vi "NI9205_UI_LinearLoadCell.vi"() -> ()   [LabVIEW 2020]
uses:
  TYPEDEF/NI9205_TD_QueueSaveData.ctl
  TYPEDEF/NI9205_TD_Method.ctl
panel:
  out "LastSaved":string
  in  "MaximumSampleRate?":bool
  in  "SampleRate":dbl=1000.0 format="%0.2f"
  out "queueDataToSave":refnum<queue>
  in  "ClearData":bool
  in  "Save Now":bool
  out "Data size":i32
  in  "Nomefile_txt":string
  in  "file path":path
  out "Meter [kN]":dbl(knob) scale=0.0..100.0
  out "Waveform Graph 2":dbl[](graph)
  out "V":dbl
  out "LC (kN)":dbl
  in  "q":dbl=2.15875
  in  "gain":dbl=-22.26172
  out "Waveform Graph":waveform(dbl)[](graph)
  in  "Stop":bool
  in  "Start":bool
  in  "Number of Samples":i32=100
  in  "Channels NI9205":tag="cDAQ2Mod2/ai6"
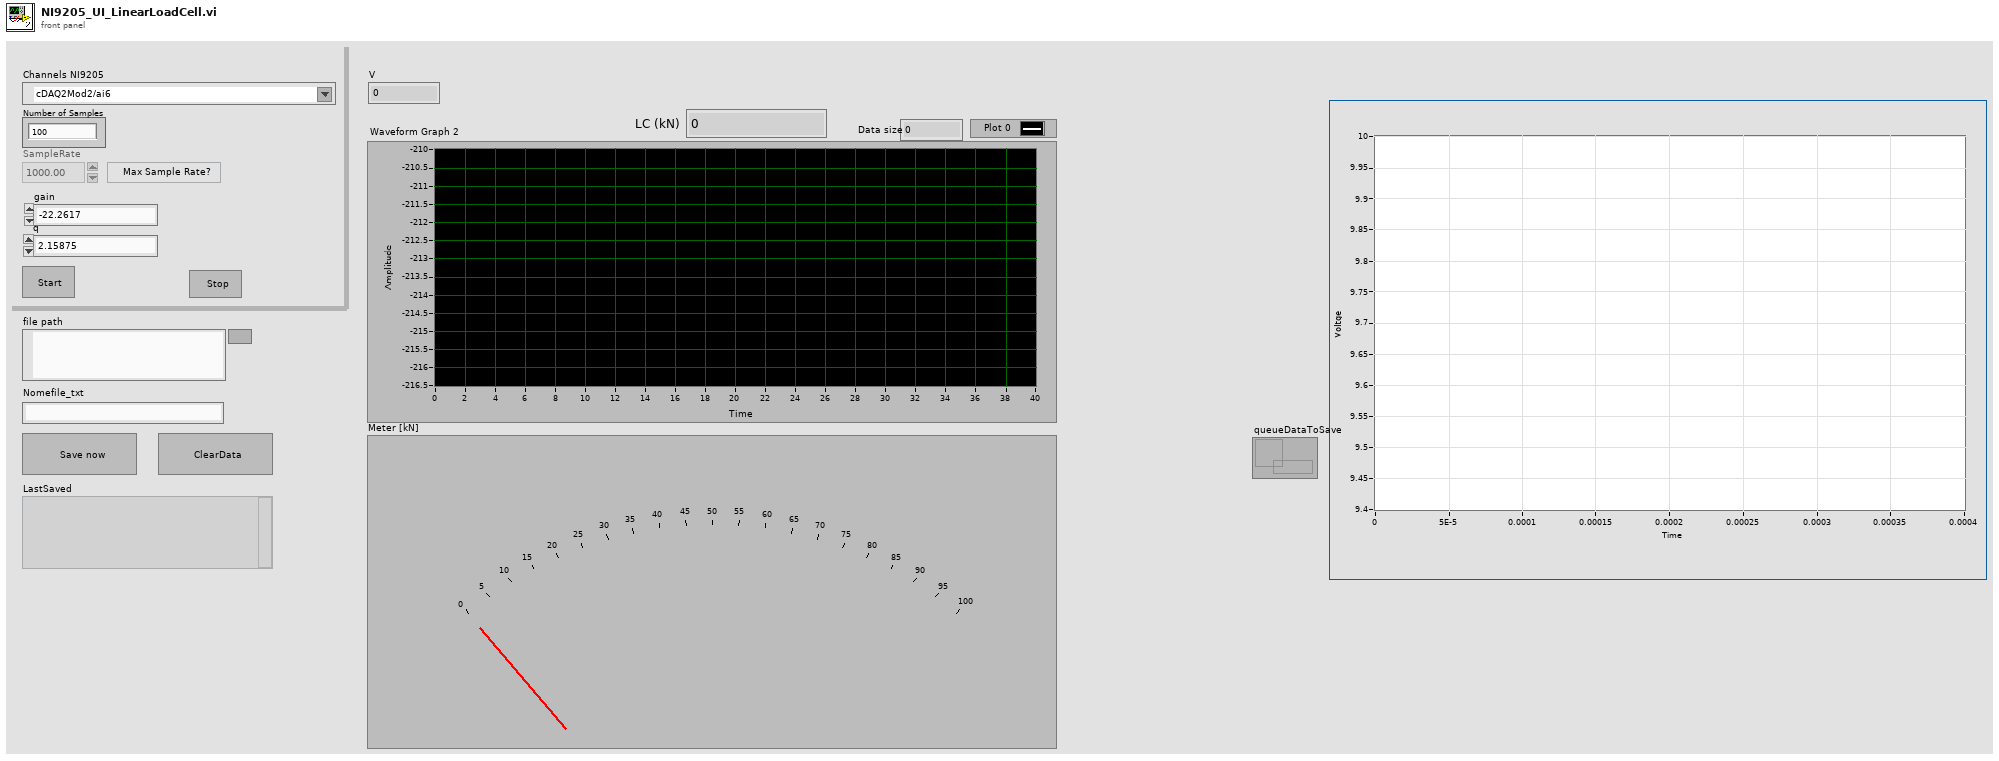
[diagram p1: front panel]
types:
  T1 = enum8{"Enabled", "Disabled", "Disabled and Grayed Out"}
  T2 = typedef "NI9205_TD_QueueSaveData.ctl" = cluster{"TimeData":timestamp[], "Ydata":dbl[], "AutoSaved?":bool}
  T3 = typedef "NI9205_TD_Method.ctl" = enum16{"NO_OP", "INIT", "SET", "GET", "CLOSE"}
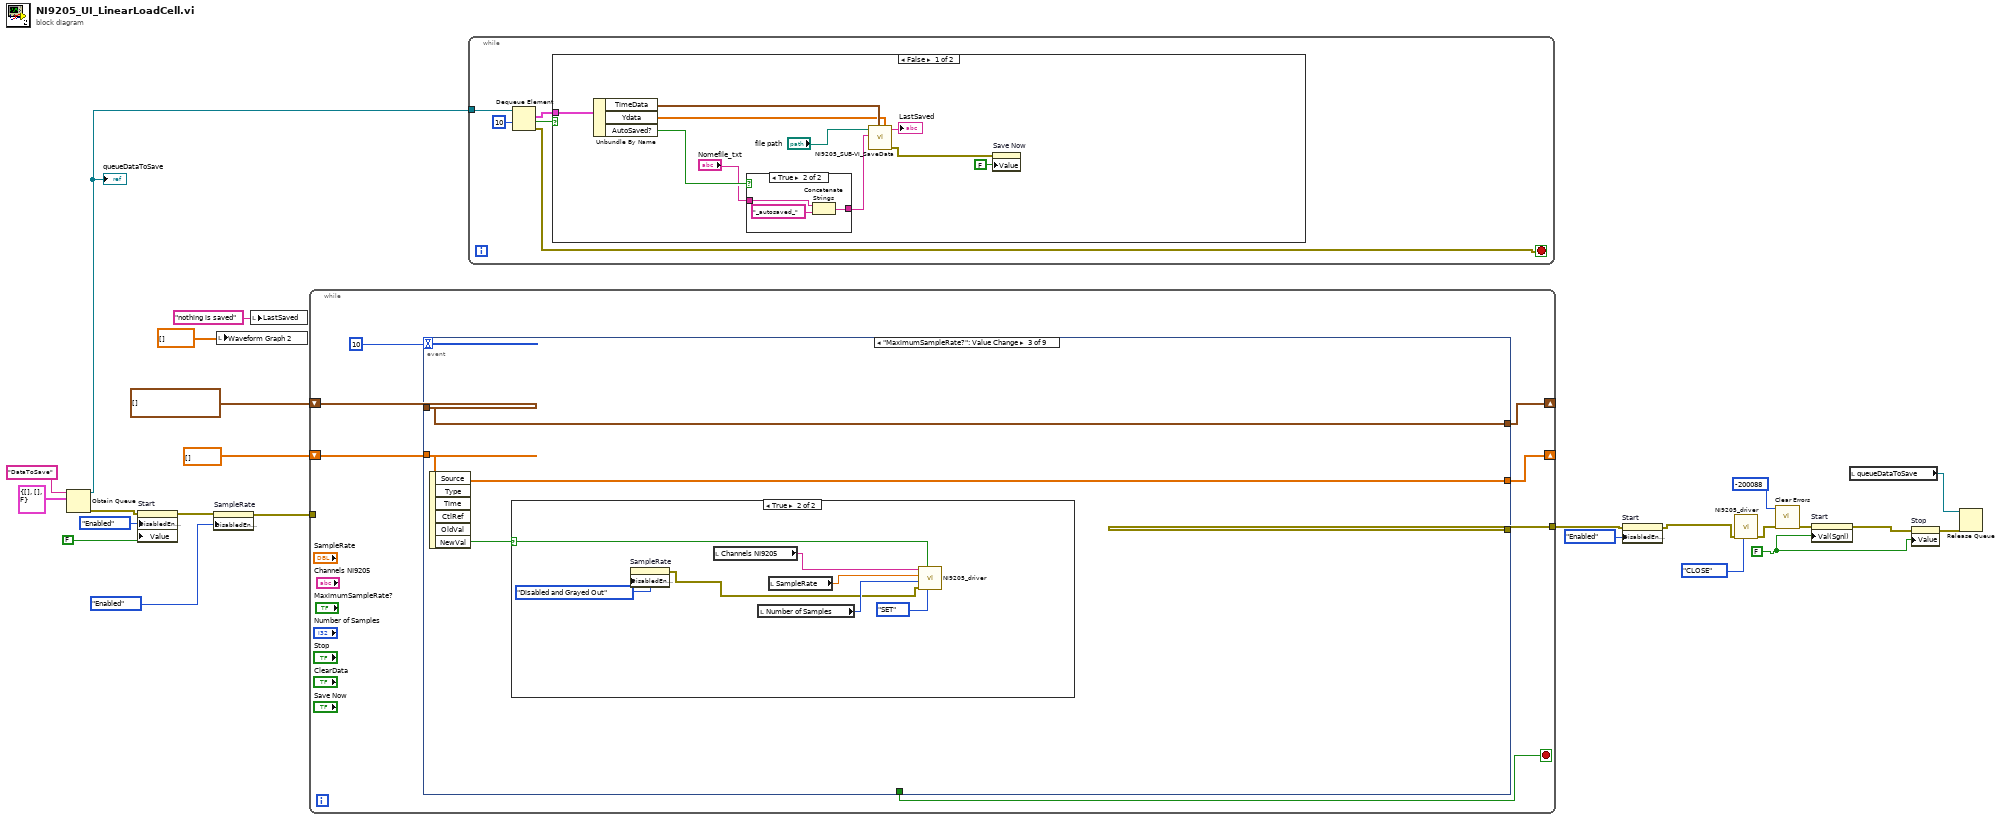
[diagram p0: block diagram]
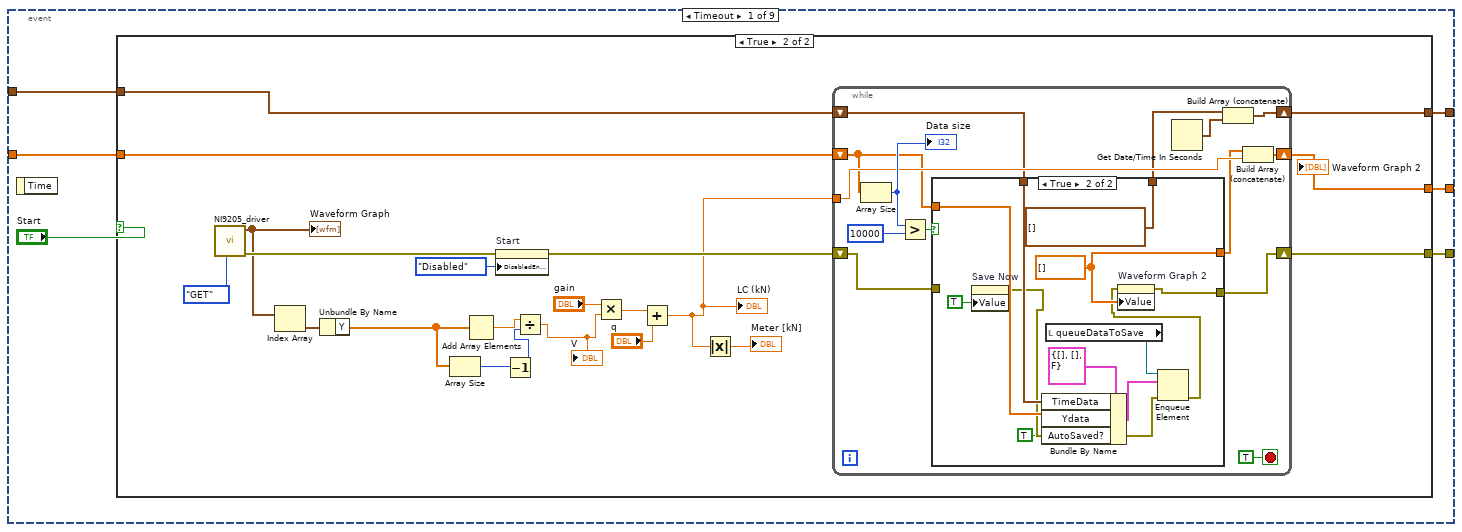
[diagram p4: hidden frame]
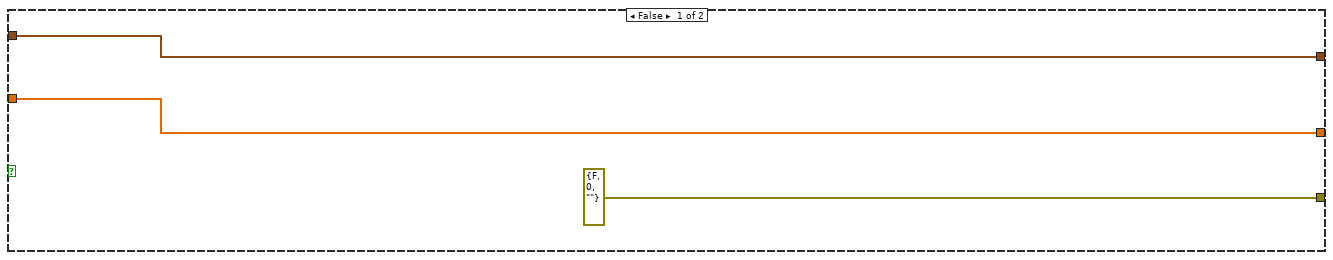
[diagram p5: hidden frame]
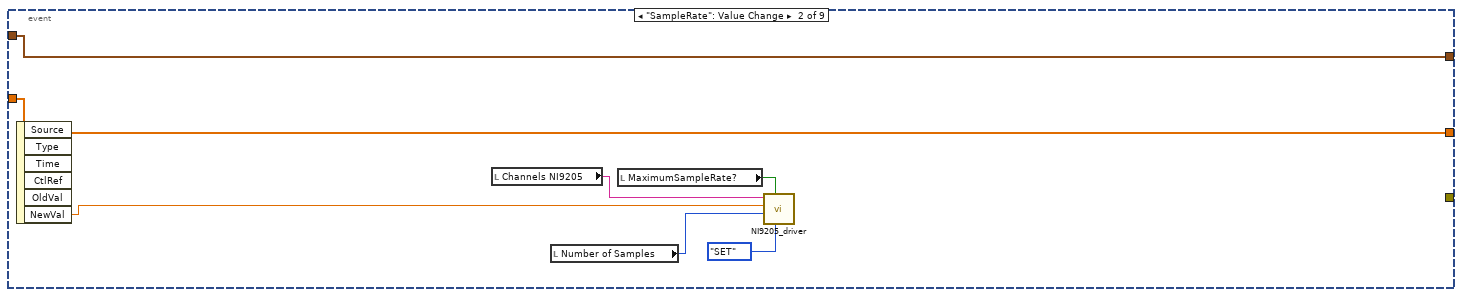
[diagram p7: hidden frame]
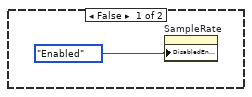
[diagram p8: hidden frame]
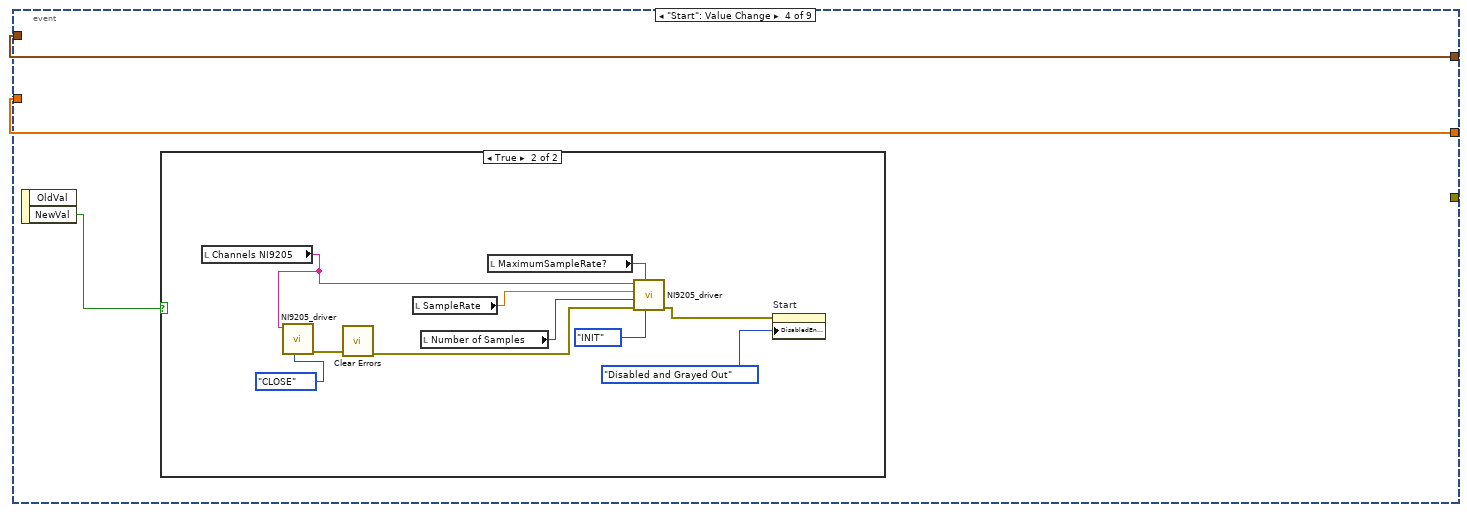
[diagram p9: hidden frame]
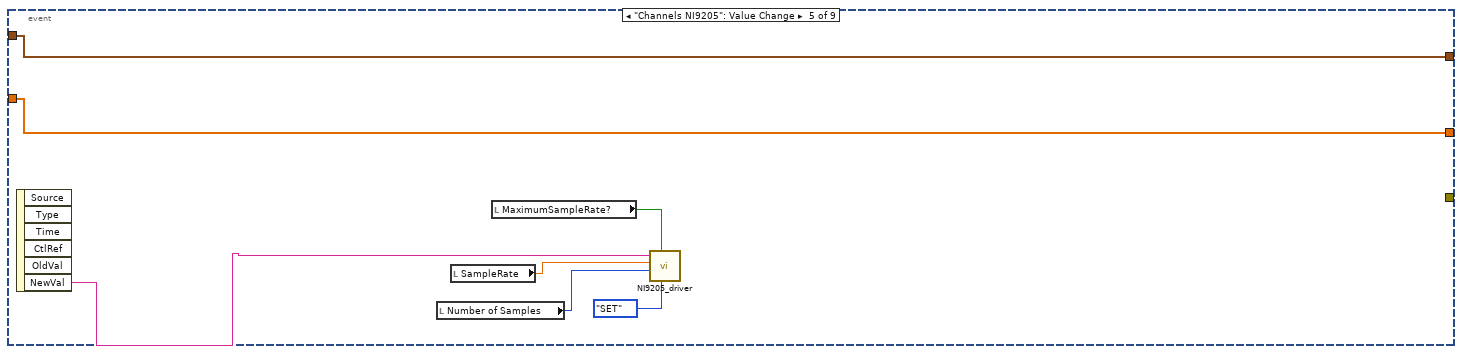
[diagram p11: hidden frame]
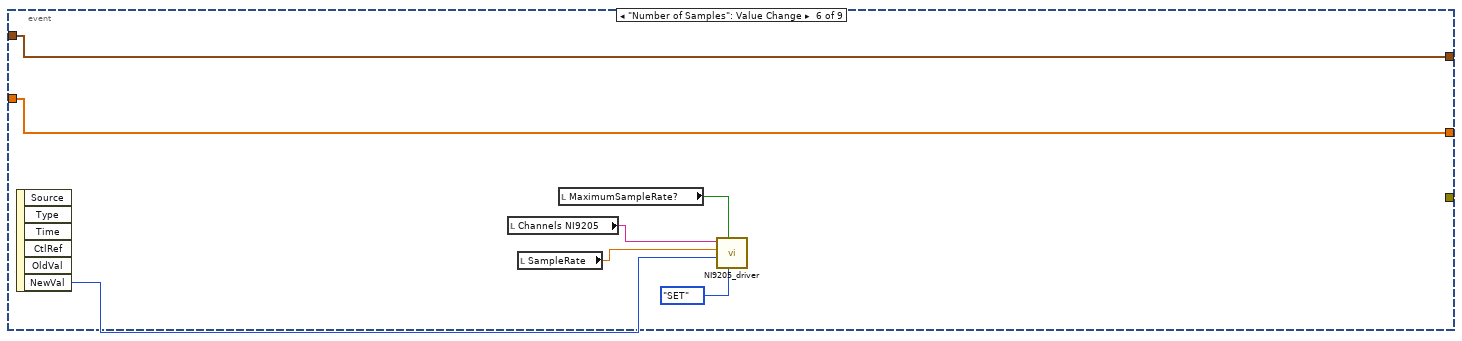
[diagram p12: hidden frame]
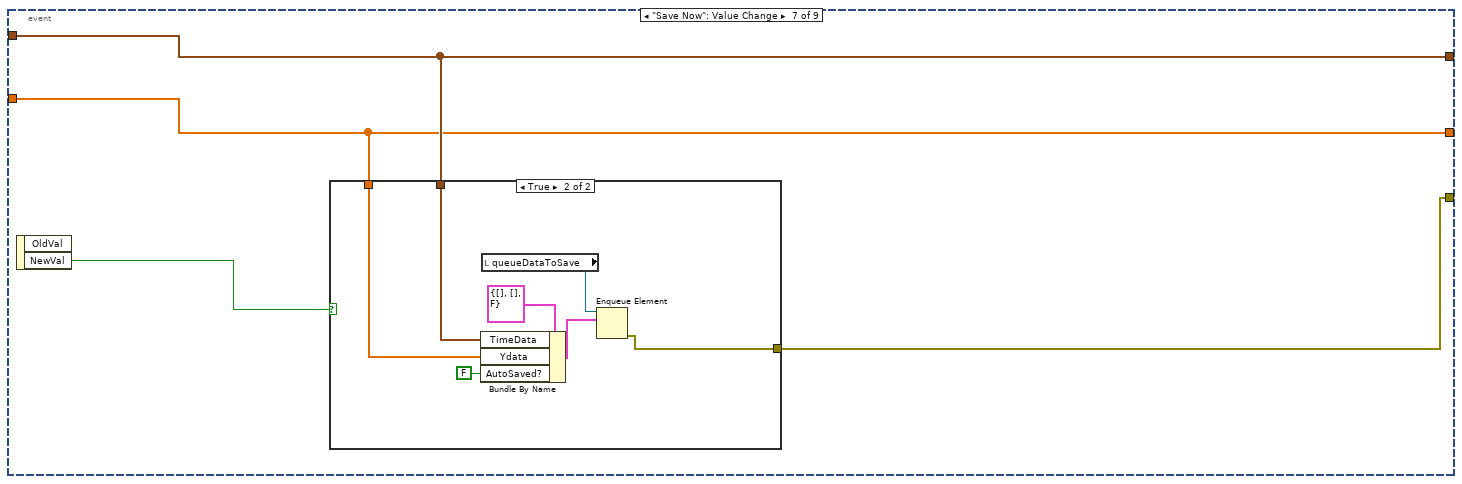
[diagram p13: hidden frame]
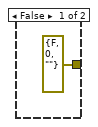
[diagram p14: hidden frame]
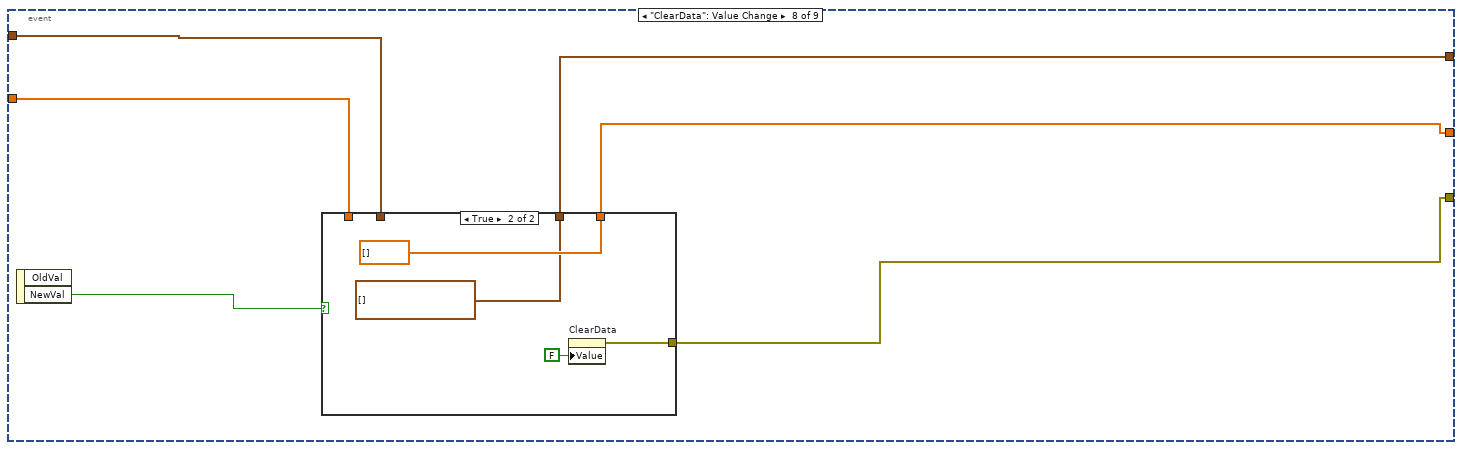
[diagram p15: hidden frame]
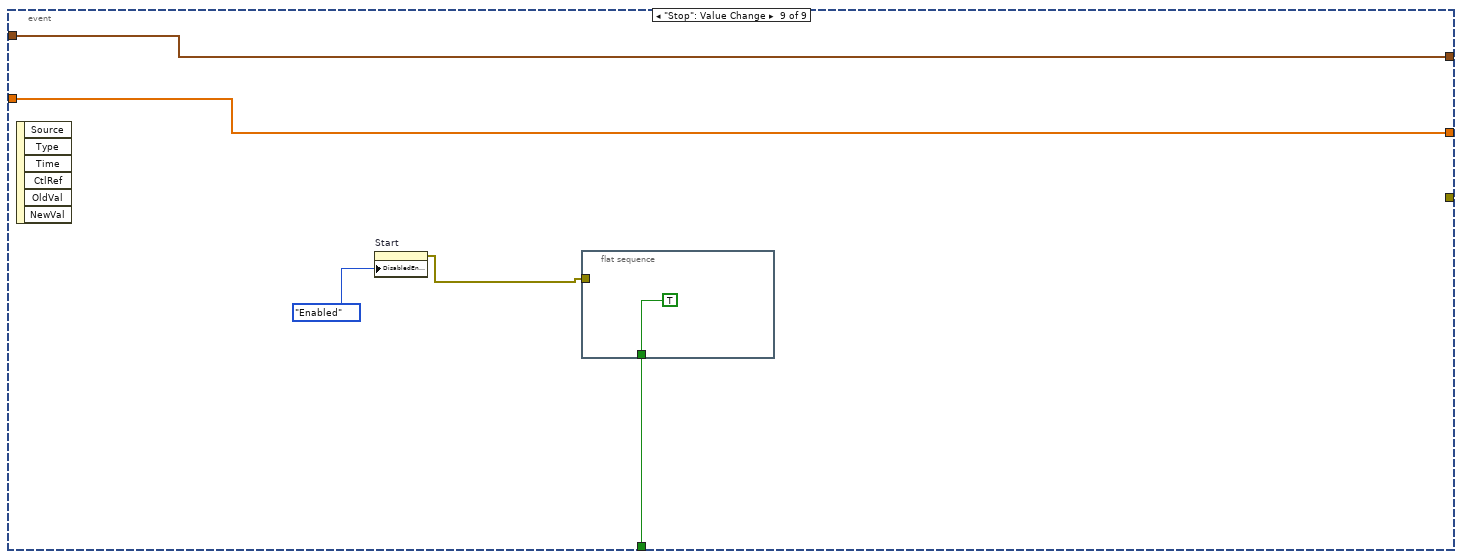
[diagram p17: hidden frame]
diagram:
  w19 = FALSE
  n1 = Obtain Queue(name (unnamed)="DataToSave", element data type=T2 {"TimeData"=[], "Ydata"=[], "AutoSaved?"=FALSE} ("DataToSave")) -> (queue out=w12:refnum<queue>, error out=w8:errorcluster)  [unwired: 3 in, 1 out]
  "queueDataToSave" <- w12
  n2 = property on="Start" class="Bool (strict)"(error in=w8, "DisabledEnum"=T1."Enabled" ("Disabled"), "Value"=FALSE ("Start")) -> (error out=w2:errorcluster)  [unwired: 1 in, 1 out]
  n3 = property on="SampleRate" class="DigNum (strict)"(error in=w2, "DisabledEnum"=T1."Enabled" ("Disabled")) -> (error out=w1:errorcluster)  [unwired: 1 in, 1 out]
  n4 = local write "Waveform Graph 2"(dbl[] []) -> ()
  n5 = local write "LastSaved"("nothing is saved" ("LastSaved")) -> ()
  n6 = while {
    tunnel: [w31] -> w23
    shift-right: [w27] -> _
    shift-left: dbl[] [] -> [w28]
    shift-right: [w25] -> _
    shift-left: timestamp[] [] -> [w26]
    tunnel: w1 -> [_]
    stop <- w30 stop-if-true
    n7 = event shown="[2] \"MaximumSampleRate?\": Value Change" {
      selector: _ -> [_ _ _ _ _ _ _ _ _]
      dyn-events: _ -> [_ _ _ _ _ _ _ _ _]
      timeout: 10 -> [_ _ _ _ _ _ _ _ _]
      tunnel: [w36 _ _ _ _ _ w136 w148 _] -> w31
      tunnel: [_ _ _ _ _ _ _ _ w164] -> w30
      tunnel: w28 -> [w35 w97 w100 w111 w128 w135 w137 w149 w163]
      tunnel: [w34 w97 w100 w111 w128 w135 w137 w152 w163] -> w27
      tunnel: [w33 w96 w99 w110 w127 w134 w138 w151 w162] -> w25
      tunnel: w26 -> [w32 w96 w99 w110 w127 w134 w138 w150 w162]
      event Timeout {
        n8 = event-data() -> ()  [unwired: 1 in, 1 out]
        n9 = case shown="True" "Start" {
          tunnel: [errorcluster {"status"=FALSE, "code"=0, "source"=""} ("error out") w51] -> w36
          tunnel: w35 -> [w39 w49]
          tunnel: [w39 w48] -> w34
          tunnel: [w38 w47] -> w33
          tunnel: w32 -> [w38 w46]
          frame False {
          }
          frame True {
            n10 = call "NI9205_driver.vi"("Method NI9205"=NI9205_TD_Method."GET") -> ("error out"=w60:errorcluster, "Waveform Graph"=w58:waveform(dbl)[])  [unwired: 8 in, 1 out]
            "Waveform Graph" <- w58
            n11 = Index Array(array=w58) -> (element=w57:waveform(dbl))  [unwired: 1 in]
            n12 = Unbundle By Name(w57) -> ("Y"=w45:dbl[])
            n13 = Array Size(array=w45) -> (size(s)=w44:i32)
            n14 = Add Array Elements(numeric array=w45) -> (sum=w43:dbl)
            n15 = property on="Start" class="Bool (strict)"(error in=w60, "DisabledEnum"=T1."Disabled" ("Disabled")) -> (error out=w52:errorcluster)  [unwired: 1 in, 1 out]
            n16 = Decrement(x=w44) -> (x-1=w42:i32)
            n17 = Divide(x=w43, y=w42) -> (x/y=w41:dbl)
            "V" <- w41
            n18 = Multiply(x="gain", y=w41) -> (x*y=w55:dbl)
            n19 = Add(x=w55, y="q") -> (x+y=w50:dbl)
            "LC (kN)" <- w50
            n20 = Absolute Value(x=w50) -> (abs(x)=→"Meter [kN]":dbl)
            n21 = while {
              shift-right: [w73] -> w51
              shift-left: w52 -> [w63]
              tunnel: w50 -> [w72]
              shift-right: [w71] -> w48
              shift-left: w49 -> [w68]
              shift-right: [w66] -> w47
              shift-left: w46 -> [w65]
              stop <- TRUE stop-if-true
              n22 = Array Size(array=w68) -> (size(s)=w75:i32)
              "Data size" <- w75
              n23 = Greater?(x=w75, y=10000) -> (0:w74:bool)
              n24 = case shown="True" w74 {
                tunnel: w63 -> [w78 _]
                tunnel: [w78 w82] -> w73
                tunnel: w68 -> [w77 w85]
                tunnel: [w77 w90] -> w70
                tunnel: w65 -> [w76 w86]
                tunnel: [w76 timestamp[] []] -> w64
                frame False {
                }
                frame True {
                  w90 = dbl[] [] ("Waveform Graph 2")
                  n25 = property on="Save Now" class="Bool (strict)"("Value"=TRUE ("Save Now")) -> (error out=w80:errorcluster)  [unwired: 2 in, 1 out]
                  n26 = Bundle By Name(cluster=T2 {"TimeData"=[], "Ydata"=[], "AutoSaved?"=FALSE} ("DataToSave"), "TimeData"=w86, "Ydata"=w85, "AutoSaved?"=TRUE) -> (w84:T2)
                  n27 = local read "queueDataToSave"() -> (w88:refnum<queue>)
                  n28 = Enqueue Element(queue=w88, element=w84, error in (no error)=w80) -> (error out=w83:errorcluster)  [unwired: 1 in, 2 out]
                  n29 = property on="Waveform Graph 2" class="WFGraph (strict)"(error in=w83, "Value"=w90) -> (error out=w82:errorcluster)  [unwired: 1 in, 1 out]
                }
              }
              n30 = Get Date/Time In Seconds() -> (seconds since 1Jan1904=w67:timestamp)
              n31 = Build Array (concatenate)(w64, w67) -> (w66:timestamp[])
              n32 = Build Array (concatenate)(w70, w72) -> (w71:dbl[])
            }
            "Waveform Graph 2" <- w48
          }
        }
      }
      event "SampleRate": Value Change {
        n33 = event-data() -> ("NewVal"=w91:dbl)  [unwired: 1 in, 5 out]
        n34 = local read "Channels NI9205"() -> (w95:tag)
        n35 = local read "Number of Samples"() -> (w92:i32)
        n36 = local read "MaximumSampleRate?"() -> (w93:bool)
        n37 = call "NI9205_driver.vi"("Method NI9205"=NI9205_TD_Method."SET", "MaximumSampleRate?"=w93, "Number of Samples"=w92, "SampleRate"=w91, "Channels NI9205"=w95) -> ()  [unwired: 4 in, 3 out]
      }
      event "MaximumSampleRate?": Value Change {
        n38 = event-data() -> ("NewVal"=w98:bool)  [unwired: 1 in, 5 out]
        n39 = case shown="True" w98 {
          selector: w98 -> [_ w104]
          frame False {
            n40 = property on="SampleRate" class="DigNum (strict)"("DisabledEnum"=T1."Enabled" ("Disabled")) -> ()  [unwired: 2 in, 2 out]
          }
          frame True {
            n41 = property on="SampleRate" class="DigNum (strict)"("DisabledEnum"=T1."Disabled and Grayed Out" ("Disabled")) -> (error out=w102:errorcluster)  [unwired: 2 in, 1 out]
            n42 = local read "Channels NI9205"() -> (w108:tag)
            n43 = local read "Number of Samples"() -> (w106:i32)
            n44 = local read "SampleRate"() -> (w107:dbl)
            n45 = call "NI9205_driver.vi"("Method NI9205"=NI9205_TD_Method."SET", "MaximumSampleRate?"=w104, "error in (no error)"=w102, "Number of Samples"=w106, "SampleRate"=w107, "Channels NI9205"=w108) -> ()  [unwired: 3 in, 3 out]
          }
        }
      }
      event "Start": Value Change {
        n46 = event-data() -> ("NewVal"=w109:bool)  [unwired: 1 in, 1 out]
        n47 = case shown="True" w109 {
          frame False {
          }
          frame True {
            n48 = local read "Channels NI9205"() -> (w114:tag)
            n49 = call "NI9205_driver.vi"("Method NI9205"=NI9205_TD_Method."CLOSE", "Channels NI9205"=w114) -> ("error out"=w117:errorcluster)  [unwired: 7 in, 2 out]
            n50 = call <vilib>:"Clear Errors.vi"("error in (no error)"=w117) -> ("error out"=w115:errorcluster)  [unwired: 5 in, 1 out]
            n51 = local read "SampleRate"() -> (w118:dbl)
            n52 = local read "Number of Samples"() -> (w120:i32)
            n53 = local read "MaximumSampleRate?"() -> (w121:bool)
            n54 = call "NI9205_driver.vi"("Method NI9205"=NI9205_TD_Method."INIT", "MaximumSampleRate?"=w121, "error in (no error)"=w115, "Number of Samples"=w120, "SampleRate"=w118, "Channels NI9205"=w114) -> ("error out"=w112:errorcluster)  [unwired: 3 in, 2 out]
            n55 = property on="Start" class="Bool (strict)"(error in=w112, "DisabledEnum"=T1."Disabled and Grayed Out" ("Disabled")) -> ()  [unwired: 1 in, 2 out]
          }
        }
      }
      event "Channels NI9205": Value Change {
        n56 = event-data() -> ("NewVal"=w122:tag)  [unwired: 1 in, 5 out]
        n57 = local read "Number of Samples"() -> (w123:i32)
        n58 = local read "SampleRate"() -> (w124:dbl)
        n59 = local read "MaximumSampleRate?"() -> (w125:bool)
        n60 = call "NI9205_driver.vi"("Method NI9205"=NI9205_TD_Method."SET", "MaximumSampleRate?"=w125, "Number of Samples"=w123, "SampleRate"=w124, "Channels NI9205"=w122) -> ()  [unwired: 4 in, 3 out]
      }
      event "Number of Samples": Value Change {
        n61 = event-data() -> ("NewVal"=w129:i32)  [unwired: 1 in, 5 out]
        n62 = local read "Channels NI9205"() -> (w130:tag)
        n63 = local read "SampleRate"() -> (w131:dbl)
        n64 = local read "MaximumSampleRate?"() -> (w132:bool)
        n65 = call "NI9205_driver.vi"("Method NI9205"=NI9205_TD_Method."SET", "MaximumSampleRate?"=w132, "Number of Samples"=w129, "SampleRate"=w131, "Channels NI9205"=w130) -> ()  [unwired: 4 in, 3 out]
      }
      event "Save Now": Value Change {
        n66 = event-data() -> ("NewVal"=w139:bool)  [unwired: 1 in, 1 out]
        n67 = case shown="True" w139 {
          tunnel: w138 -> [_ w144]
          tunnel: w137 -> [_ w143]
          tunnel: [errorcluster {"status"=FALSE, "code"=0, "source"=""} ("error out") w142] -> w136
          frame False {
          }
          frame True {
            n68 = Bundle By Name(cluster=T2 {"TimeData"=[], "Ydata"=[], "AutoSaved?"=FALSE} ("DataToSave"), "TimeData"=w144, "Ydata"=w143, "AutoSaved?"=FALSE) -> (w146:T2)
            n69 = local read "queueDataToSave"() -> (w147:refnum<queue>)
            n70 = Enqueue Element(queue=w147, element=w146) -> (error out=w142:errorcluster)  [unwired: 2 in, 2 out]
          }
        }
      }
      event "ClearData": Value Change {
        n71 = event-data() -> ("NewVal"=w153:bool)  [unwired: 1 in, 1 out]
        n72 = case shown="True" w153 {
          tunnel: [w154 dbl[] []] -> w152
          tunnel: [w155 timestamp[] []] -> w151
          tunnel: w150 -> [w155 _]
          tunnel: w149 -> [w154 _]
          tunnel: [_ w156] -> w148
          frame False {
          }
          frame True {
            n73 = property on="ClearData" class="Bool (strict)"("Value"=FALSE ("ClearData")) -> (error out=w156:errorcluster)  [unwired: 2 in, 1 out]
          }
        }
      }
      event "Stop": Value Change {
        n74 = event-data() -> ()  [unwired: 1 in, 6 out]
        n75 = property on="Start" class="Bool (strict)"("DisabledEnum"=T1."Enabled" ("Disabled")) -> (error out=w160:errorcluster)  [unwired: 2 in, 1 out]
        n76 = flat-sequence {
          tunnel: [TRUE] -> w164
          tunnel: w160 -> [_]
          frame #0 {
          }
        }
      }
    }
  }
  n77 = while {
    tunnel: w12 -> [w170]
    stop <- w166 stop-if-true
    n78 = Dequeue Element(queue=w170, timeout in ms (-1)=10) -> (element=w167:T2, timed out?=w168:bool, error out=w166:errorcluster)  [unwired: 1 in, 1 out]
    n79 = case shown="False" w168 {
      tunnel: w167 -> [w180 _]
      frame False {
        n80 = Unbundle By Name(w180) -> ("TimeData"=w179:timestamp[], "Ydata"=w178:dbl[], "AutoSaved?"=w173:bool)
        n81 = case shown="True" w173 {
          tunnel: "Nomefile_txt" -> [w181 w184]
          tunnel: [w181 w182] -> w171
          frame False {
          }
          frame True {
            n82 = Concatenate Strings(w184, "_autosaved_" ("string")) -> (w182:string)
          }
        }
        n83 = call "NI9205_SUB-VI_SaveData.vi"("Arraych6"=w178, "Array Time"=w179, "Suffisso"=w171, "file path (use dialog)"="file path") -> ("error out"=w174:errorcluster, "LastSaved"=→"LastSaved":string)  [unwired: 6 in]
        n84 = property on="Save Now" class="Bool (strict)"(error in=w174, "Value"=FALSE ("Save Now")) -> ()  [unwired: 1 in, 2 out]
      }
      frame True {
      }
    }
  }
  n85 = property on="Start" class="Bool (strict)"(error in=w23, "DisabledEnum"=T1."Enabled" ("Disabled")) -> (error out=w21:errorcluster)  [unwired: 1 in, 1 out]
  n86 = call "NI9205_driver.vi"("Method NI9205"=NI9205_TD_Method."CLOSE", "error in (no error)"=w21) -> ("error out"=w7:errorcluster)  [unwired: 7 in, 2 out]
  n87 = call <vilib>:"Clear Errors.vi"("error in (no error)"=w7, "specific error code to clear (0: all)"=-200088) -> ("error out"=w5:errorcluster)  [unwired: 4 in, 1 out]
  n88 = property on="Start" class="Bool (strict)"(error in=w5, "Val(Sgnl)"=w19) -> (error out=w20:errorcluster)  [unwired: 1 in, 1 out]
  n89 = local read "queueDataToSave"() -> (w10:refnum<queue>)
  n90 = property on="Stop" class="Bool (strict)"(error in=w20, "Value"=w19) -> (error out=w11:errorcluster)  [unwired: 1 in, 1 out]
  n91 = Release Queue(queue=w10, error in (no error)=w11) -> ()  [unwired: 1 in, 3 out]
